vi "Check Streams.vi"(8 "error in (no error)":errorcluster, 11 "PXImc Transceiver in":refnum<class "DSF PXImc Transceiver.lvclass">=refnum) -> (0 "error out":errorcluster, 3 "PXImc Transceiver out":refnum<class "DSF PXImc Transceiver.lvclass">)   [LabVIEW 2017, in "DSF Core.lvlib" / "DSF PXImc Transceiver.lvclass"]
uses:
  DSF PXImc Transceiver.lvclass
  Duplicate Stream ID Error.vi
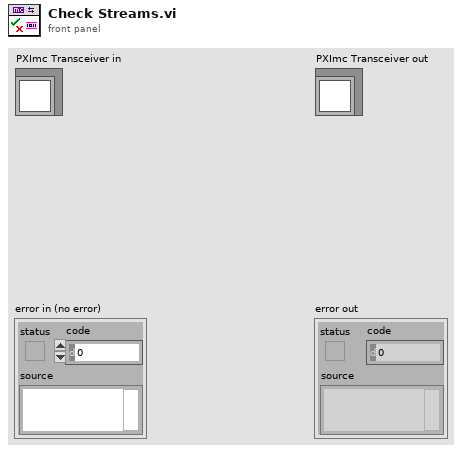
[diagram p1: front panel]
types:
  T1 = typedef "DSF Core.lvlib/DSF PXImc Transceiver.lvclass/PXImc Transfer Data.ctl" = cluster{"stream id":u16, "session":refnum<k21>, "buffer size":u64}
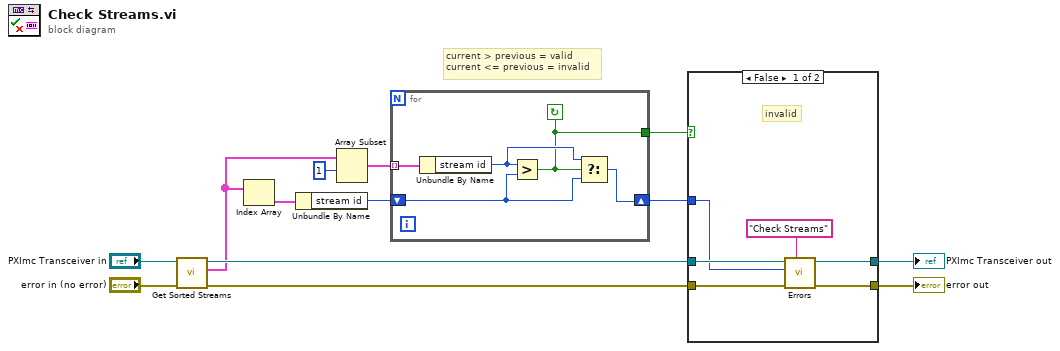
[diagram p0: block diagram]
diagram:
  # "current > previous = valid\ncurrent <= previous = invalid"
  n1 = call "Get Sorted Streams.vi"("error in (no error)"="error in (no error)", "PXImc Transceiver in"="PXImc Transceiver in") -> ("error out"=w3:errorcluster, "stream-sorted transfers"=w1:T1[], "PXImc Transceiver out"=w5:refnum<class "DSF PXImc Transceiver.lvclass">)  [unwired: 7 in]
  n2 = Index Array(array=w1) -> (element=w11:T1)  [unwired: 1 in]
  n3 = Unbundle By Name(w11) -> ("stream id"=w10:u16)
  n4 = Array Subset(array=w1, index=1) -> (w8:T1[])  [unwired: 1 in]
  n5 = for {
    tunnel: w8 -> [w18] mode=indexing
    shift-right: [w15] -> w6
    shift-left: w10 -> [w16]
    tunnel: [w14] -> w7
    stop <- w14 continue-if-true
    n6 = Unbundle By Name(w18) -> ("stream id"=w17:u16)
    n7 = Greater?(x=w17, y=w16) -> (0:w14:bool)
    n8 = Select(t=w17, s=w14, f=w16) -> (s? t:f=w15:u16)
  }
  n9 = case shown="False" w7 {
    tunnel: w3 -> [w24 w26]
    tunnel: [w23 w26] -> w2
    tunnel: w6 -> [w20 _]
    tunnel: w5 -> [w22 w25]
    tunnel: [w21 w25] -> w4
    frame False {
      # "invalid"
      n10 = call-poly "Errors.vi"("vi name"="Check Streams", "error in (no error)"=w24, "stream id"=w20, "PXImc Transceiver in"=w22) -> ("error out"=w23:errorcluster, "PXImc Transceiver out"=w21:refnum<class "DSF PXImc Transceiver.lvclass">)  [unwired: 6 in]
    }
    frame True {
      # "valid"
    }
  }
  "error out" <- w2
  "PXImc Transceiver out" <- w4
